vi "Configure Bandwidth.vi"(8 "error in (no error)":errorcluster, 10 "Bandwidth (3: off: 30MHz)":i32(ring)=3 items=["high: 30MHz", "medium: 15MHz", "low: 5MHz", "off: 30MHz"], 11 "VISA resource name":refnum<visa-resource-name>) -> (0 "error out":errorcluster, 3 "VISA resource name out":refnum<visa-resource-name>)   [LabVIEW 2018, in "Agilent U2000 Series.lvlib"]
doc: "Sets the bandwidth of the device.\n\nNote:\nThis VI supports Agilent models U2021/2XA and U2042XA/U2044XA/U2049XA only."
uses:
  Agilent U2000 Series.lvlib
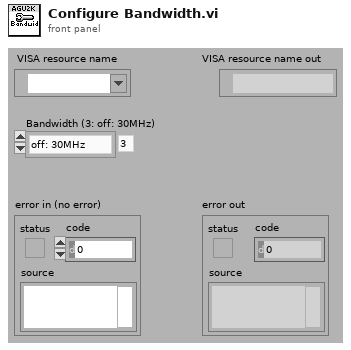
[diagram p1: front panel]
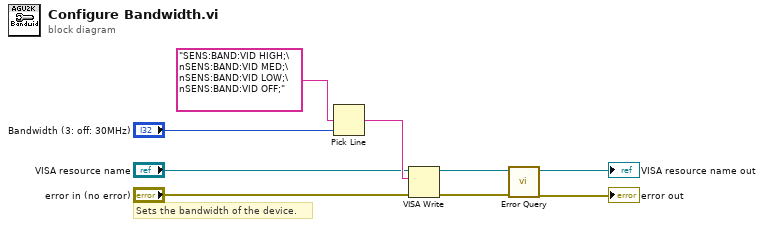
[diagram p0: block diagram]
diagram:
  # "Sets the bandwidth of the device."
  n1 = Pick Line(multi-line string="SENS:BAND:VID HIGH;\nSENS:BAND:VID MED;\nSENS:BAND:VID LOW;\nSENS:BAND:VID OFF;", line index="Bandwidth (3: off: 30MHz)") -> (output string=w7:string)  [unwired: 1 out]
  n2 = VISA Write(VISA resource name="VISA resource name", write buffer=w7, error in (no error)="error in (no error)") -> (VISA resource name out=w4:refnum<visa-resource-name>, error out=w3:errorcluster)  [unwired: 1 out]
  n3 = call "Error Query.vi"("error in (no error)"=w3, "VISA resource name"=w4) -> ("error out"=→"error out":errorcluster, "VISA resource name out"=→"VISA resource name out":refnum<visa-resource-name>)  [unwired: 8 out]
